vi "Rename Table.vi"(8 "error in":errorcluster, 9 "New Table Name":string, 10 "Existing Table Name":string, 11 "Data.PG":refnum<class "LV-Data.PGSQL.lvclass">) -> (0 "error out":errorcluster, 2 "SQL":string, 3 "Data.PG out":refnum<class "LV-Data.PGSQL.lvclass">)   [LabVIEW 2019, in "LV-Data.PGSQL.lvclass"]
uses:
  LV-Data.PGSQL.lvclass
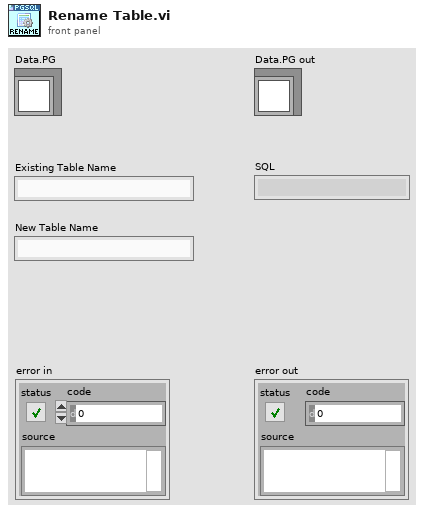
[diagram p1: front panel]
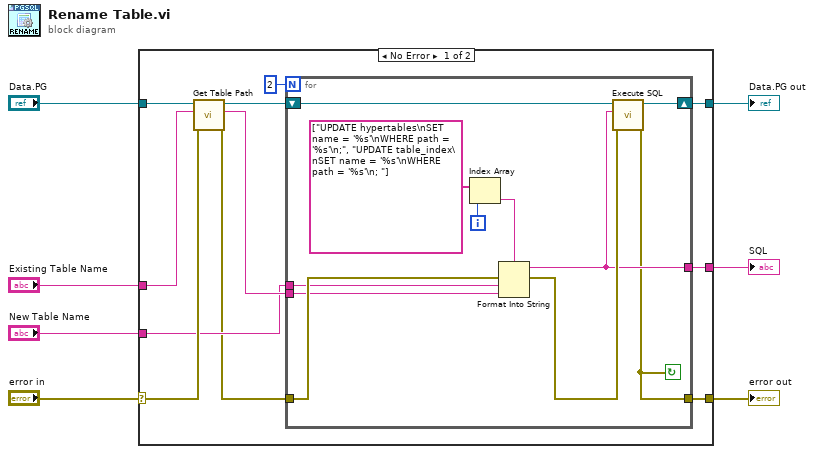
[diagram p0: block diagram]
diagram:
  n1 = case shown="No Error" "error in" {
    selector: "error in" -> [w14 w30]
    tunnel: "Existing Table Name" -> [w15 _]
    tunnel: "New Table Name" -> [w10 _]
    tunnel: [w18 _] -> w5
    tunnel: [w17 w30] -> w4
    tunnel: "Data.PG" -> [w13 w31]
    tunnel: [w16 w31] -> w2
    frame No Error {
      n2 = call "Get Table Path.vi"("error in (no error)"=w14, "Table Name"=w15, "Data.PG"=w13) -> ("error out"=w8:errorcluster, "Table Path"=w11:string, "Data.PG out"=w12:refnum<class "LV-Data.PGSQL.lvclass">)  [unwired: 5 in, 1 out]
      n3 = for {
        N: 2 -> [_]
        tunnel: w11 -> [w24]
        shift-right: [w27] -> w16
        shift-left: w12 -> [w25]
        tunnel: w8 -> [w26]
        tunnel: [w19] -> w17
        tunnel: w10 -> [w23]
        tunnel: [w28] -> w18
        i -> [w20]
        stop <- w19 continue-if-true
        n4 = Index Array(array=string[] ["UPDATE hypertables\nSET name = '%s'\nWHERE path = '%s'\n;", "UPDATE table_index\nSET name = '%s'\nWHERE path = '%s'\n; "], index=w20) -> (element=w21:string)
        n5 = Format Into String(format string=w21, error in=w26, w23, w24) -> (resulting string=w28:string, error out=w29:errorcluster)  [unwired: 1 in]
        n6 = call "Execute SQL.vi"("error in"=w29, "SQL"=w28, "LV-Data.PGSQL"=w25) -> ("error out"=w19:errorcluster, "LV-Data.PGSQL out"=w27:refnum<class "LV-Data.PGSQL.lvclass">)  [unwired: 5 in, 2 out]
      }
    }
    frame Error {
    }
  }
  "SQL" <- w5
  "error out" <- w4
  "Data.PG out" <- w2
